vi "SegmentRead.vi"(2 "error in":errorcluster, 3 "Byte Array":u8[](array[numeric]), 4 "Input Message":T1={"Timestamp(4)"=0, "Sequence(4)"=0, "JY61ACC(2)"=[], "JY61GRY(3)"=[], "JY61AGL(3)"=[], "GY52ACC(2)"=[], "GY52GRY(3)"=[], "ADC1(3)"=[], "ADC2(3)"=[], "LFT/RAT"="DIR"}) -> (0 "error out":errorcluster, 1 "Output Message":T1={"Timestamp(4)"=0, "Sequence(4)"=0, "JY61ACC(2)"=[], "JY61GRY(3)"=[], "JY61AGL(3)"=[], "GY52ACC(2)"=[], "GY52GRY(3)"=[], "ADC1(3)"=[], "ADC2(3)"=[], "LFT/RAT"="DIR"})   [LabVIEW 2014]
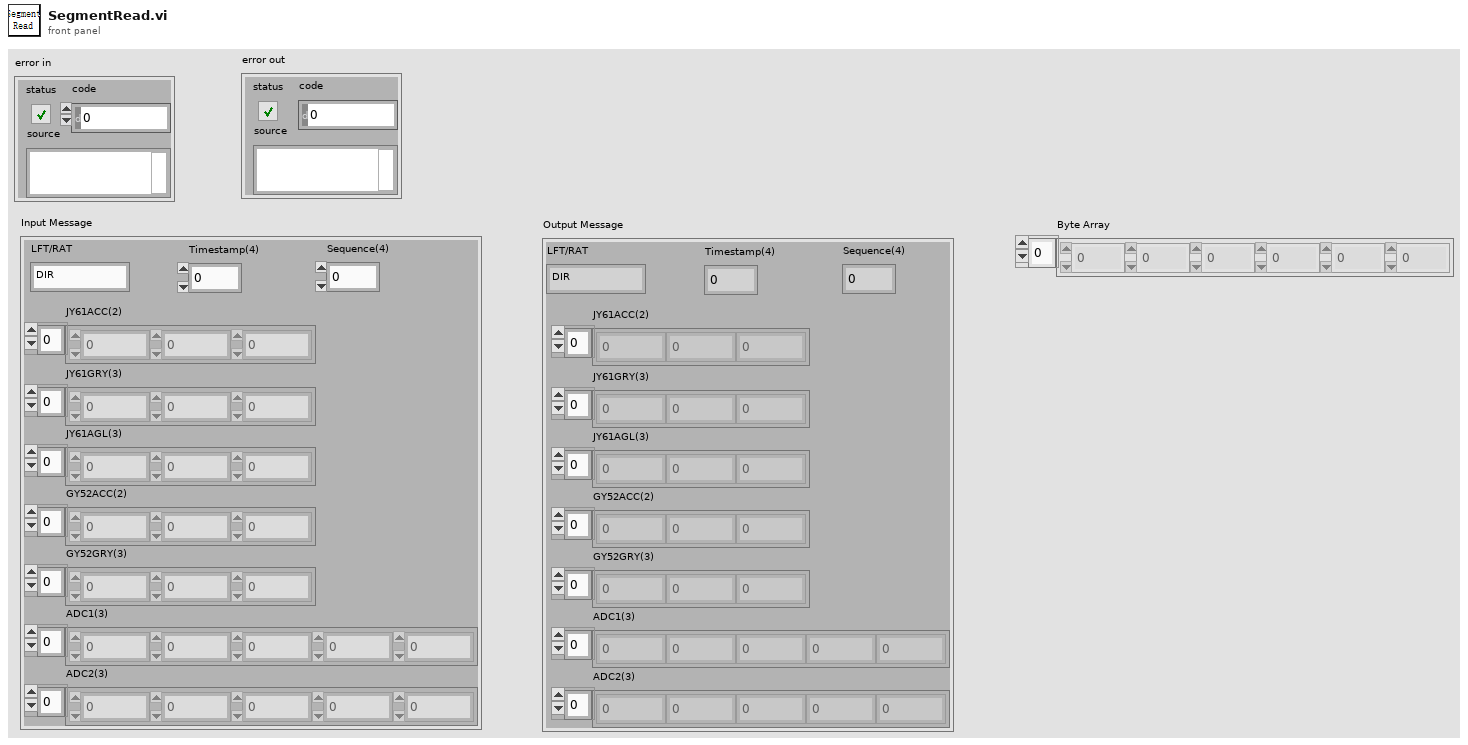
[diagram p1: front panel]
types:
  T1 = cluster{"Timestamp(4)":u32, "Sequence(4)":u32, "JY61ACC(2)":dbl[], "JY61GRY(3)":dbl[], "JY61AGL(3)":dbl[], "GY52ACC(2)":dbl[], "GY52GRY(3)":dbl[], "ADC1(3)":dbl[], "ADC2(3)":dbl[], "LFT/RAT":string}
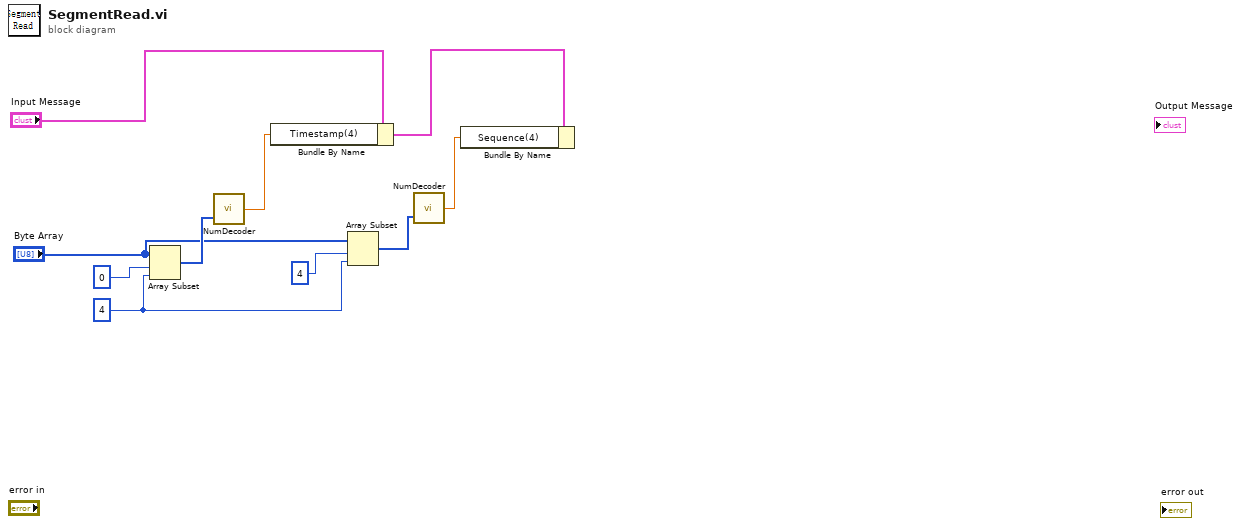
[diagram p0: block diagram]
diagram:
  w1 = 4 ("Length")
  n1 = Array Subset(array="Byte Array", index=0, length=w1) -> (w7:u8[])
  n2 = call "NumDecoder.vi"("Byte Array"=w7) -> ("Number"=w6:dbl)  [unwired: 1 in]
  n3 = Bundle By Name(cluster="Input Message", "Timestamp(4)"=w6) -> (w10:T1)
  n4 = Array Subset(array="Byte Array", index=4, length=w1) -> (w3:u8[])
  n5 = call "NumDecoder.vi"("Byte Array"=w3) -> ("Number"=w2:dbl)  [unwired: 1 in]
  n6 = Bundle By Name(cluster=w10, "Sequence(4)"=w2) -> ()  [unwired: 1 out]
